vi "main_myRIO.vi"() -> ()   [LabVIEW 2017]
uses:
  <vilib>/Platform/TimedLoop/XDataNode/timing_clust.ctl
  <vilib>/Platform/TimedLoop/XDataNode/nitl_modes.ctl
  <vilib>/Platform/TimedLoop/XDataNode/wakeup.ctl
  <vilib>/myRIO/Instrument Drivers/Onboard IO/DIO/typedefs/DIO Reference.ctl
  <vilib>/myRIO/Common/Instrument Driver Framework/Utilities/typedefs/myRIO Generic Hardware Reference.ctl
  <vilib>/myRIO/Common/Instrument Driver Framework/Utilities/typedefs/Hardware Version Enum.ctl
  <vilib>/myRIO/Common/Instrument Driver Framework/Utilities/typedefs/myRIO v1.0 Reference.ctl
  <vilib>/myRIO/Common/Instrument Driver Framework/Utilities/typedefs/Generic FPGA Reference.ctl
  <vilib>/myRIO/Common/Instrument Driver Framework/myRIO v1.0/DIO/typedefs/DIO Channels List.ctl
  <vilib>/myRIO/Common/Instrument Driver Framework/myRIO v1.0/DIO/typedefs/DIO Channels Enum.ctl
  <vilib>/userdefined/High Color/nirio_resource_hc.ctl
  <vilib>/myRIO/Instrument Drivers/Onboard IO/PWM/typedefs/PWM Reference.ctl
  <vilib>/myRIO/Common/Instrument Driver Framework/myRIO v1.0/PWM/typedefs/PWM Channels Enum.ctl
  <vilib>/myRIO/Instrument Drivers/Onboard IO/PWM/typedefs/PWM Configuration.ctl
  <vilib>/myRIO/Common/Instrument Driver Framework/Utilities/vis/Is FPGA Ref Available.vi
  <vilib>/myRIO/Common/Instrument Driver Framework/myRIO v1.0/DIO/vis/myRIO v1.1 Open DIO.vi
  <vilib>/myRIO/Instrument Drivers/Onboard IO/DIO/vis/Write.vi
  <vilib>/myRIO/Common/Instrument Driver Framework/myRIO v1.0/PWM/vis/myRIO v1.1 Open PWM.vi
  <vilib>/myRIO/Instrument Drivers/Onboard IO/PWM/vis/Set Duty Cycle and Frequency.vi
  <vilib>/myRIO/Common/Instrument Driver Framework/Utilities/vis/Validate Channels.vi
  <vilib>/myRIO/Common/Instrument Driver Framework/myRIO v1.0/DIO/vis/myRIO v1.0 Reserve DIO.vi
  <vilib>/myRIO/Common/Instrument Driver Framework/myRIO v1.0/PWM/vis/myRIO v1.0 Reserve PWM.vi
  <vilib>/myRIO/Common/Instrument Driver Framework/myRIO v1.0/UART/vis/myRIO v1.0 Close UART.vi
  <vilib>/myRIO/Common/Instrument Driver Framework/myRIO v1.0/Resource Manager/vis/myRIO v1.0 Reserve Channel List.vi
  <vilib>/myRIO/Common/Instrument Driver Framework/myRIO v1.0/DIO/vis/myRIO v1.0 Build MUX Configuration DIO.vi
  <vilib>/myRIO/Common/Instrument Driver Framework/myRIO v1.0/PWM/vis/myRIO v1.0 Build MUX Configuration PWM.vi
  <vilib>/myRIO/Common/Instrument Driver Framework/myRIO v1.0/Resource Manager/vis/myRIO v1.0 Reserve Channel.vi
  <vilib>/myRIO/Common/Instrument Driver Framework/myRIO v1.0/Resource Manager/vis/myRIO v1.0 Unreserve Channel.vi
  <vilib>/myRIO/Common/Instrument Driver Framework/myRIO v1.0/Resource Manager/vis/myRIO v1.0 Create Configuration List.vi
  <vilib>/myRIO/Common/Instrument Driver Framework/myRIO v1.0/Resource Manager/vis/myRIO v1.0 Build Mutex Name.vi
  <vilib>/Utility/VariantDataType/GetNumericInfo.vi
  <vilib>/Utility/error.llb/Error Cluster From Error Code.vi
  <vilib>/myRIO/Common/Instrument Driver Framework/myRIO v1.0/myRIO v1.1 Open.vi
  <vilib>/myRIO/Common/Instrument Driver Framework/Utilities/vis/IO Manager.vi
  <vilib>/myRIO/Common/Instrument Driver Framework/Utilities/vis/Configuration Manager.vi
  <vilib>/myRIO/Common/Instrument Driver Framework/myRIO v1.0/Resource Manager/vis/myRIO v1.0 Configure IO.vi
  <vilib>/myRIO/Common/Instrument Driver Framework/myRIO v1.0/myRIO v1.0 Close.vi
  <vilib>/myRIO/Common/Instrument Driver Framework/myRIO v1.0/DIO/vis/myRIO v1.0 Write DIO.vi
  <vilib>/myRIO/Common/Instrument Driver Framework/myRIO v1.0/PWM/vis/myRIO v1.0 Write PWM.vi
  <vilib>/myRIO/Common/Instrument Driver Framework/Utilities/vis/FPGA Ref Manager.vi
  <vilib>/myRIO/Common/Instrument Driver Framework/myRIO v1.0/myRIO v1.0 Reset FPGA.vi
  <vilib>/myRIO/Common/Instrument Driver Framework/myRIO v1.0/IRQ/vis/myRIO v1.0 IRQ Info FGV.vi
  <vilib>/myRIO/Common/Instrument Driver Framework/myRIO v1.0/IRQ/vis/myRIO v1.0 Timer IRQ Info FGV.vi
  <vilib>/myRIO/Common/Instrument Driver Framework/myRIO v1.0/IRQ/vis/myRIO v1.0 ISR Agent.vi
  <vilib>/platform/TimedLoop/XDataNode/XDataNode.xnode
  <vilib>/myRIO/Express VI/Onboard IO/DO/DO Express VI.xnode
  <vilib>/myRIO/Instrument Drivers/Onboard IO/DIO/vis/myRIO DIO Open.xnode
  <vilib>/myRIO/Express VI/Onboard IO/PWM/PWM Express VI.xnode
  <vilib>/myRIO/Instrument Drivers/Onboard IO/PWM/vis/myRIO PWM Open.xnode
  <vilib>/Platform/TimedLoop/XDataNode/XDNodeRunTimeDep.lvlib
  <vilib>/myRIO/Instrument Drivers/Utilities/Utilities.lvlib
  <vilib>/myRIO/Instrument Drivers/Onboard IO/PWM/PWM.lvlib
  <vilib>/myRIO/Instrument Drivers/Onboard IO/DIO/DIO.lvlib
panel:
  out "Stop program":bool
  out "speed":i64
  out "Finished Late":bool
  out "reset frame":bool
  out "X duty Cycle":dbl
  out "Y duty Cycle":dbl
  out "Array":cluster{dbl, dbl, bool}[](array[cluster])
  out "maxYServo":dbl
  out "minYServo":dbl
  out "maxXServo":dbl
  out "minXServo":dbl
  out "maxY":dbl
  out "minY":dbl
  out "maxX":dbl
  out "minX":dbl
  out "Frequency":dbl
  in  "Stop myRIO":bool
  # "myRIO debugging interface"
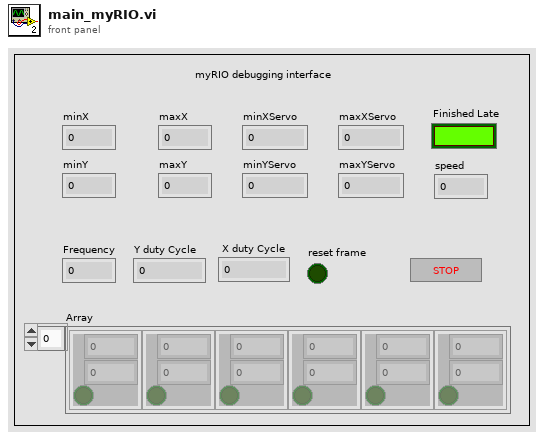
[diagram p1: front panel]
types:
  T1 = typedef "DIO.lvlib/DIO Reference.ctl" = cluster{"myRIO Reference":T2, "DIO Channels List":T6}
  T2 = typedef "myRIO Generic Hardware Reference.ctl" = cluster{"myRIO Model":T3, "myRIO Hardware Reference":T4}
  T3 = typedef "Hardware Version Enum.ctl" = enum16{"Unknown", "myRIO-1900", "myRIO-1950", "roboRIO", "NI ELVIS RIO CM"}
  T4 = typedef "myRIO v1.0 Reference.ctl" = cluster{"Generic FPGA Reference":T5, "Allow multiple opens":bool}
  T5 = typedef "Generic FPGA Reference.ctl" = refnum<k20>
  T6 = typedef "DIO Channels List.ctl" = T7[]
  T7 = typedef "DIO Channels Enum.ctl" = enum16{"Not Connected", "C/DIO0", "C/DIO1", "C/DIO2", "C/DIO3", "C/DIO4", "C/DIO5", "C/DIO6", "C/DIO7", "A/DIO0", "A/DIO1", "A/DIO2", "A/DIO3", "A/DIO4", "A/DIO5", "A/DIO6", "A/DIO7", "A/DIO8", "A/DIO9", "A/DIO10", "A/DIO11", "A/DIO12", "A/DIO13", "A/DIO14", "A/DIO15", "B/DIO0", "B/DIO1", "B/DIO2", "B/DIO3", "B/DIO4", "B/DIO5", "B/DIO6", "B/DIO7", "B/DIO8", "B/DIO9", "B/DIO10", "B/DIO11", "B/DIO12", "B/DIO13", "B/DIO14", "B/DIO15", "LED0", "LED1", "LED2", "LED3", "Button0", "DIO/DIO0", "DIO/DIO1", "DIO/DIO2", "DIO/DIO3", "DIO/DIO4", "DIO/DIO5", "DIO/DIO6", "DIO/DIO7", "DIO/DIO8", "DIO/DIO9", "SPI/CS0", "SPI/CS1", "SPI/CS2", "SPI/CS3", "LED RADIO (Green)", "LED RADIO (Red)", "LED COMM (Green)", "LED COMM (Red)", "LED MODE (Green)", "LED MODE (Red)"}
  T8 = typedef "nirio_resource_hc.ctl" = tag
  T9 = typedef "PWM.lvlib/PWM Reference.ctl" = cluster{"myRIO Reference":T2, "PWM Channels Enum":T10, "PWM Configuration":T11}
  T10 = typedef "PWM Channels Enum.ctl" = enum16{"Not Connected", "C/PWM0", "C/PWM1", "A/PWM0", "A/PWM1", "A/PWM2", "B/PWM0", "B/PWM1", "B/PWM2", "PWM/PWM0", "PWM/PWM1", "PWM/PWM2", "PWM/PWM3", "PWM/PWM4", "PWM/PWM5", "PWM/PWM6", "PWM/PWM7", "PWM/PWM8", "PWM/PWM9"}
  T11 = typedef "PWM.lvlib/PWM Configuration.ctl" = cluster{"Frequency":dbl, "Duty Cycle":dbl}
  T12 = typedef "XDNodeRunTimeDep.lvlib/timing_clust.ctl" = cluster{"Expected End [f-1]":u64, "Actual End [f-1]":u64, "Finished Late? [f-1]":bool, "Expected End [i-1]":u64, "Actual End [i-1]":u64, "Finished Late? [i-1]":bool, "Expected Start [i]":u64, "Actual Start [i]":u64, "Expected Start [f]":u64, "Actual Start [f]":u64, "Source Name":string, "Structure Name":string, "Period":i64, "Deadline":i64, "Offset":i64, "Start":i64, "Priority":i32, "Timeout":i32, "Mode":T13, "Wakeup Reason":T14, "Error":errorcluster, "Source Type":string, "Secondary Source Type":string, "Global End Time":u64, "Global Start Time":u64, "Frame Duration":u64, "Iteration Duration":u64, "Assigned CPU":i32, "I/O Scan Engine Mode":u32}
  T13 = typedef "XDNodeRunTimeDep.lvlib/nitl_modes.ctl" = enum32{"No Change", "Process missed periods, maintain original phase", "Discard missed periods, maintain original phase", "Process missed periods, ignore original phase", "Discard missed periods, ignore original phase"}
  T14 = typedef "XDNodeRunTimeDep.lvlib/wakeup.ctl" = enum32{"Normal", "Aborted", "Asynchronous wakeup", "Timing source error", "Timed loop error", "Timeout"}
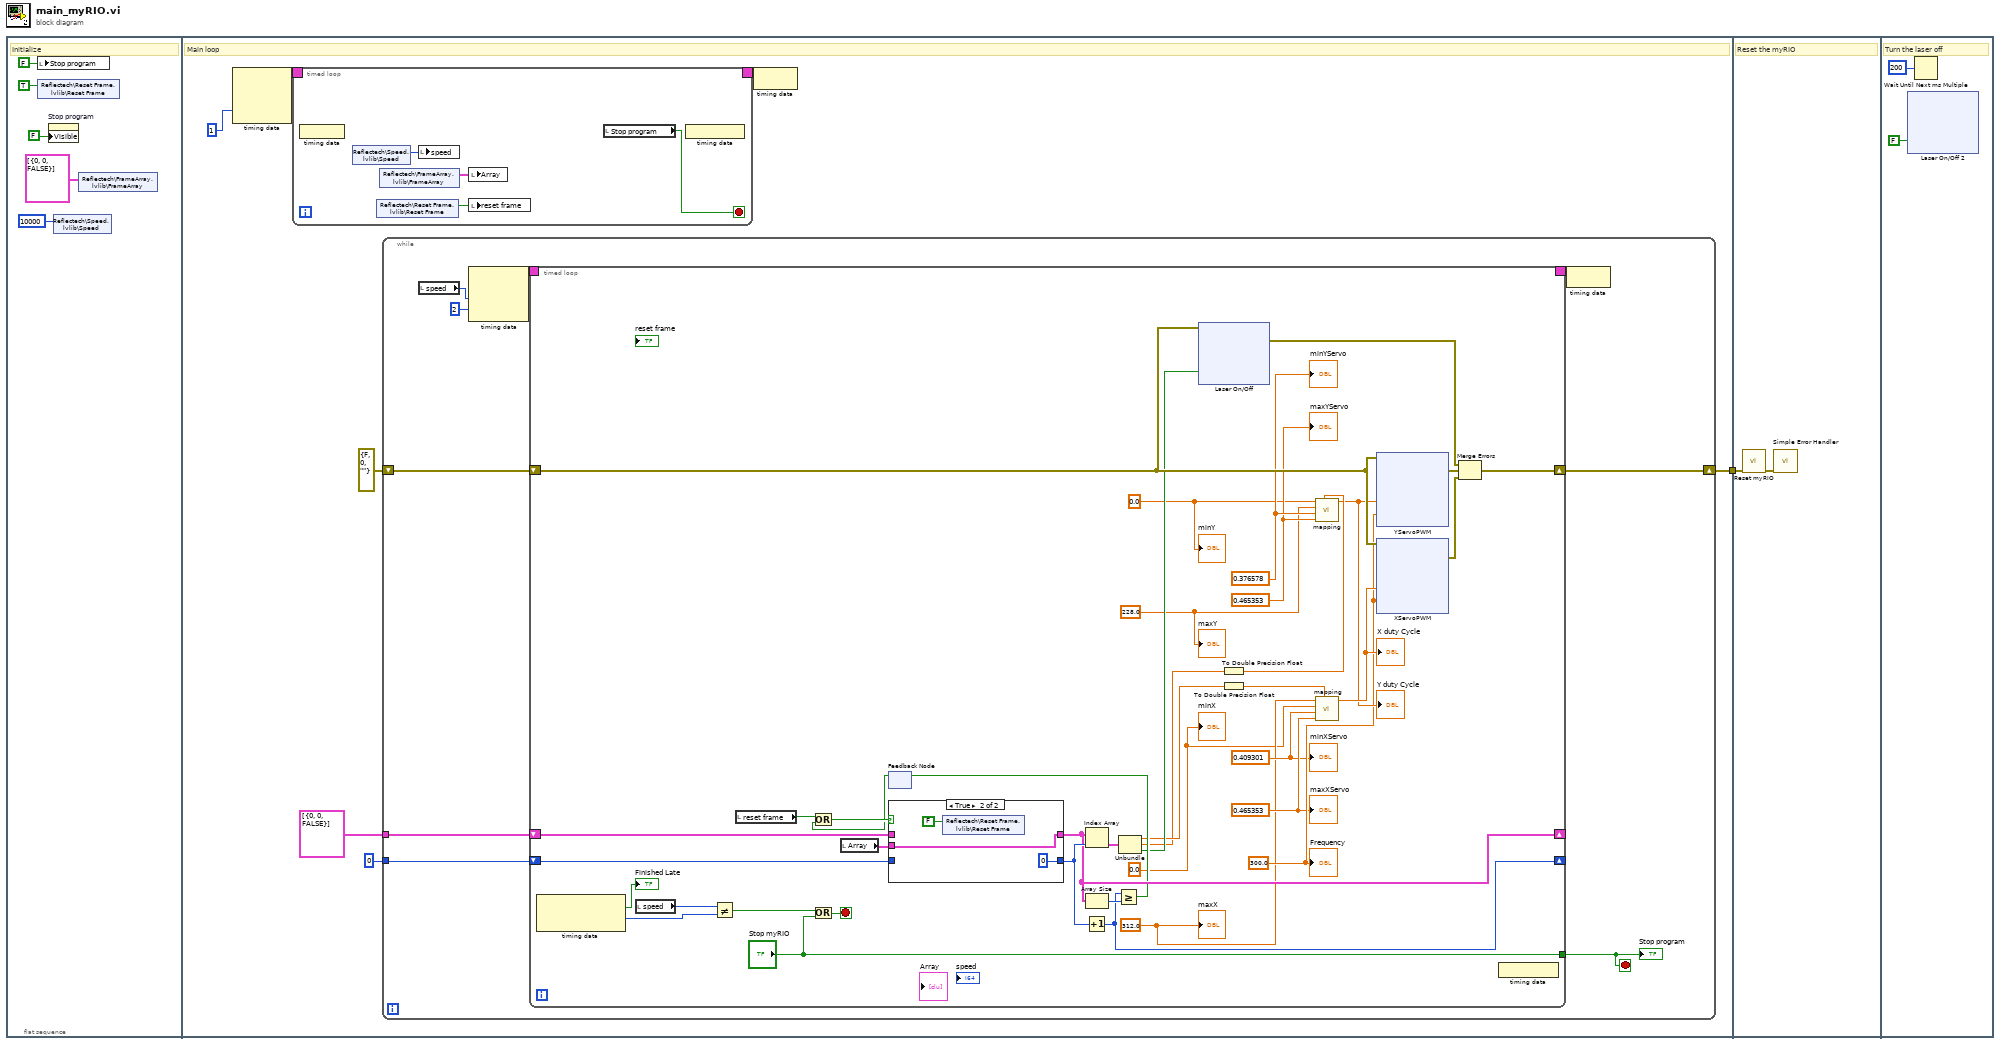
[diagram p0: block diagram]
diagram:
  n1 = flat-sequence {
    tunnel: [w13] -> w1
    tunnel: w1 -> [w191]
    frame #0 {
      # "Initialize"
      n2 = local write "Stop program"(FALSE ("Stop program")) -> ()
      n3 = shared-variable "Reflectech\\Reset Frame.lvlib\\Reset Frame"(TRUE ("Reset Frame")) -> ()  [unwired: 1 in, 1 out]
      n4 = property on="Stop program" class="Bool (strict)"("Visible"=FALSE) -> ()  [unwired: 2 in, 2 out]
      n5 = shared-variable "Reflectech\\Speed.lvlib\\Speed"(i64 10000 ("Speed")) -> ()  [unwired: 1 in, 1 out]
      n6 = shared-variable "Reflectech\\FrameArray.lvlib\\FrameArray"(cluster{i32, i32, bool}[] [{0, 0, FALSE}] ("ImageArray")) -> ()  [unwired: 1 in, 1 out]
    }
    frame #1 {
      # "Main loop"
      n7 = node-c288(1 ("Priority")) -> (w9:T12)  [unwired: 2 in]
      n8 = timed-loop {
        timing: w9 -> [_]
        timing-out: [_] -> w8
        stop <- w181 stop-if-true
        n9 = node-c288() -> ()  [unwired: 1 in]
        n10 = shared-variable "Reflectech\\Speed.lvlib\\Speed"() -> (w182:i64)  [unwired: 1 in, 1 out]
        n11 = shared-variable "Reflectech\\Reset Frame.lvlib\\Reset Frame"() -> (w183:bool)  [unwired: 1 in, 1 out]
        n12 = shared-variable "Reflectech\\FrameArray.lvlib\\FrameArray"() -> (w184:cluster{i32, i32, bool}[])  [unwired: 1 in, 1 out]
        n13 = local write "speed"(w182) -> ()
        n14 = local write "Array"(w184) -> ()
        n15 = local write "reset frame"(w183) -> ()
        n16 = local read "Stop program"() -> (w181:bool)
        n17 = node-c288() -> ()  [unwired: 1 out]
      }
      n18 = while {
        tunnel: 0 -> [w19]
        tunnel: cluster{i32, i32, bool}[] [{0, 0, FALSE}] ("ImageArray") -> [w18]
        shift-right: [w20] -> w13
        shift-left: errorcluster {"status"=FALSE, "code"=0, "source"=""} ("error in (no error)") -> [w17]
        stop <- w14 stop-if-true
        n19 = local read "speed"() -> (w15:i64)
        n20 = node-c288(w15, 2 ("Priority")) -> (w22:T12)  [unwired: 1 in]
        n21 = timed-loop {
          timing: w22 -> [_]
          timing-out: [_] -> w21
          shift-right: [w54] -> w20
          shift-left: w17 -> [w52]
          shift-right: [w53] -> _
          shift-left: w18 -> [w61]
          shift-right: [w47] -> _
          shift-left: w19 -> [w49]
          tunnel: ["Stop myRIO"] -> w14
          stop <- w26 stop-if-true
          w31 = 0.0 ("minX")
          w32 = 0.0 ("minX")
          w33 = 228.0 ("minX")
          w34 = 312.0 ("minX")
          w35 = 0.409301 ("minX")
          w36 = 0.465353 ("minX")
          w37 = 300.0 ("Frequency")
          w38 = 0.465353 ("minX")
          w39 = 0.376578 ("minX")
          n22 = node-c288() -> (→"Finished Late":bool, w24:i64)  [unwired: 1 in]
          n23 = local read "speed"() -> (w27:i64)
          n24 = Not Equal?(x=w27, y=w24) -> (x != y?=w25:bool)
          n25 = local read "reset frame"() -> (w29:bool)
          n26 = Or(x=w25, y="Stop myRIO") -> (x .or. y?=w26:bool)
          n27 = local read "Array"() -> (w30:cluster{dbl, dbl, bool}[])
          n28 = feedback #1() -> (w45:bool)  [unwired: 1 in]
          n29 = Or(x=w29, y=w45) -> (x .or. y?=w50:bool)
          n30 = case shown="True" w50 {
            tunnel: [w133 w136] -> w53
            tunnel: w30 -> [_ w136]
            tunnel: w61 -> [w133 _]
            tunnel: w49 -> [w132 _]
            tunnel: [w132 0] -> w60
            frame False {
            }
            frame True {
              n31 = shared-variable "Reflectech\\Reset Frame.lvlib\\Reset Frame"(FALSE ("Reset Frame")) -> ()  [unwired: 1 in, 1 out]
            }
          }
          n32 = Index Array(array=w53, index=w60) -> (element=w59:cluster{dbl, dbl, bool})
          n33 = Array Size(array=w53) -> (size(s)=w48:i32)
          n34 = Increment(x=w60) -> (x+1=w47:i32)
          n35 = Greater Or Equal?(x=w47, y=w48) -> (x >= y?=w46:bool)
          n36 = feedback-in #1(w46) -> ()
          n37 = Unbundle(w59) -> (w42:dbl, w41:dbl, w44:bool)
          n38 = xnode "Laser On/Off"("A/DIO1 (Pin 13)"=w44, "error in (no error)"=w52) -> ("error out"=w51:errorcluster)
          n39 = To Double Precision Float(number=w41) -> (double precision float=w57:dbl)
          n40 = To Double Precision Float(number=w42) -> (double precision float=w58:dbl)
          n41 = call "mapping.vi"("in"=w57, "maxOut"=w38, "minOut"=w39, "maxIn"=w33, "minIn"=w31) -> ("out"=w40:dbl)  [unwired: 6 in]
          "Y duty Cycle" <- w40
          n42 = call "mapping.vi"("in"=w58, "maxOut"=w36, "minOut"=w35, "maxIn"=w32, "minIn"=w34) -> ("out"=w43:dbl)  [unwired: 6 in]
          "X duty Cycle" <- w43
          n43 = xnode "YServoPWM"("Duty Cycle"=w40, "Frequency [Hz]"=w37, "error in (no error)"=w52) -> ("error out"=w56:errorcluster)
          n44 = xnode "XServoPWM"("Duty Cycle"=w43, "Frequency [Hz]"=w37, "error in (no error)"=w52) -> ("error out"=w55:errorcluster)
          n45 = Merge Errors(w51, w56, w55) -> (w54:errorcluster)
          n46 = node-c288() -> ()  [unwired: 1 out]
          "minYServo" <- w39
          "maxYServo" <- w38
          "Frequency" <- w37
          "maxXServo" <- w36
          "minXServo" <- w35
          "maxX" <- w34
          "maxY" <- w33
          "minX" <- w32
          "minY" <- w31
        }
        "Stop program" <- w14
        n47 = node-c288(w21) -> ()
      }
      n48 = node-c288(w8) -> ()
    }
    frame #2 {
      # "Reset the myRIO"
      n49 = call <vilib>:"Reset myRIO.vi"("error in (no error)"=w191) -> ("error out"=w192:errorcluster)  [unwired: 10 in]
      n50 = call <vilib>:"Simple Error Handler.vi"("error in (no error)"=w192) -> ()  [unwired: 4 in, 5 out]
    }
    frame #3 {
      # "Turn the laser off"
      n51 = xnode "Laser On/Off 2"("A/DIO1 (Pin 13)"=FALSE) -> ()  [unwired: 1 in, 1 out]
      n52 = Wait Until Next ms Multiple(millisecond multiple=u32 200) -> ()  [unwired: 1 out]
    }
  }
